vi "Read Asynchronous Measurement (Current).vi"(6 "Wait Time (10 S)":i32=10, 8 "error in (no error)":errorcluster, 9 "Current Buffer (smua.nvbuffer1)":string="smua.nvbuffer1", 10 "Source Measure Unit Channel (0: Channel A)":i32(ring) items=["Channel A", "Channel B"], 11 "VISA resource name":refnum<visa-resource-name>) -> (0 "error out":errorcluster, 2 "Current Buffer Data (A)":dbl[](array[numeric]), 3 "VISA resource name out":refnum<visa-resource-name>)   [LabVIEW 2015, in "Keithley 2600 Series.lvlib"]
doc: "Returns the asynchronous current measurements."
uses:
  Keithley 2600 Series.lvlib
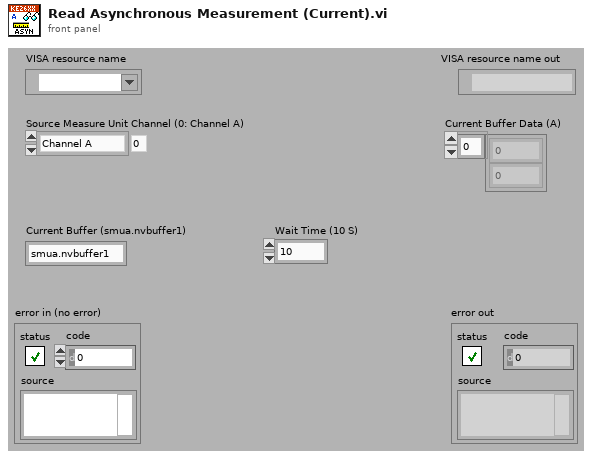
[diagram p1: front panel]
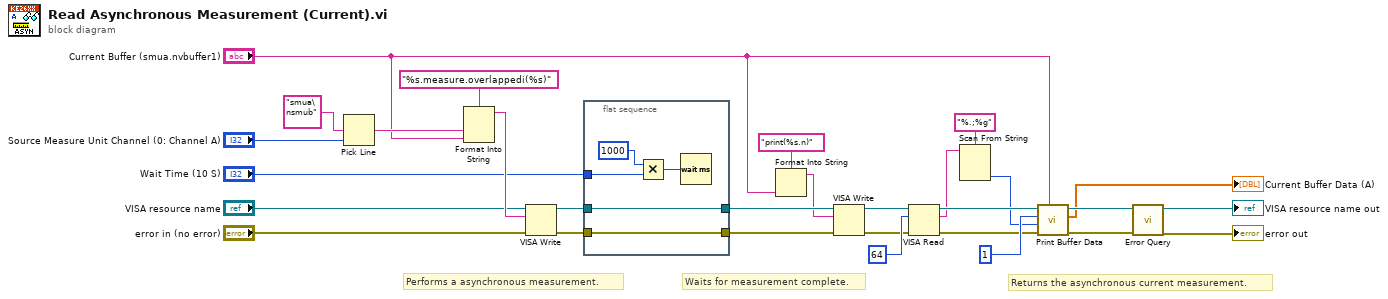
[diagram p0: block diagram]
diagram:
  # "Performs a asynchronous measurement."
  # "Waits for measurement complete."
  # "Returns the asynchronous current measurement."
  n1 = Pick Line(multi-line string="smua\nsmub", line index="Source Measure Unit Channel (0: Channel A)") -> (output string=w21:string)  [unwired: 1 in]
  n2 = Format Into String(format string="%s.measure.overlappedi(%s)", w21, "Current Buffer (smua.nvbuffer1)") -> (resulting string=w28:string)  [unwired: 2 in, 1 out]
  n3 = VISA Write(VISA resource name="VISA resource name", write buffer=w28, error in (no error)="error in (no error)") -> (VISA resource name out=w10:refnum<visa-resource-name>, error out=w9:errorcluster)  [unwired: 1 out]
  n4 = flat-sequence {
    tunnel: w10 -> [w34]
    tunnel: [w34] -> w7
    tunnel: w9 -> [w33]
    tunnel: [w33] -> w5
    tunnel: "Wait Time (10 S)" -> [w32]
    frame #0 {
      n5 = Multiply(x=1000, y=w32) -> (x*y=w30:i32)
      n6 = Wait (ms)(milliseconds to wait=w30) -> ()  [unwired: 1 out]
    }
  }
  n7 = Format Into String(format string="print(%s.n)", "Current Buffer (smua.nvbuffer1)") -> (resulting string=w2:string)  [unwired: 2 in, 1 out]
  n8 = VISA Write(VISA resource name=w7, write buffer=w2, error in (no error)=w5) -> (VISA resource name out=w6:refnum<visa-resource-name>, error out=w4:errorcluster)  [unwired: 1 out]
  n9 = VISA Read(VISA resource name=w6, byte count=u32 64, error in (no error)=w4) -> (VISA resource name out=w15:refnum<visa-resource-name>, read buffer=w13:string, error out=w14:errorcluster)  [unwired: 1 out]
  n10 = Scan From String(format string="%.;%g", input string=w13) -> (output 1=w12:i32)  [unwired: 3 in, 3 out]
  n11 = call "Print Buffer Data.vi"("Reading Buffer (smua.nvbuffer1)"="Current Buffer (smua.nvbuffer1)", "error in (no error)"=w14, "End Index (1)"=w12, "Start Index (1)"=1 ("Start Index (0)"), "VISA resource name"=w15) -> ("error out"=w18:errorcluster, "Buffer Data"=→"Current Buffer Data (A)":dbl[], "VISA resource name out"=w19:refnum<visa-resource-name>)  [unwired: 4 in]
  n12 = call "Error Query.vi"("error in (no error)"=w18, "VISA resource name"=w19) -> ("error out"=→"error out":errorcluster, "VISA resource name out"=→"VISA resource name out":refnum<visa-resource-name>)  [unwired: 6 in, 2 out]
